vi "Run Post-Compile Hook.vi"(7 "Datum":refnum<class "Datum.lvclass">, 8 "Error In":errorcluster, 10 "Hooks In":T1, 11 "Output In":string) -> (0 "Error Out":errorcluster, 2 "Hooks Out":T1, 3 "Output Out":string)   [LabVIEW 2018, in "Toolkit.lvlib"]
uses:
  Toolkit.lvlib
  Low-Level/Type Definitions/Hooks.ctl
  Hooks/Compile/Process/Process.lvclass
  Hooks/Render/Comment/Comment.lvclass
  Hooks/Render/Delimiter/Delimiter.lvclass
  Hooks/Render/Node/Node.lvclass
  Hooks/Render/Partial/Partial.lvclass
  Hooks/Render/Process/Process.lvclass
  Hooks/Render/Section/Section.lvclass
  Hooks/Render/Text/Text.lvclass
  Hooks/Render/Variable/Variable.lvclass
  Data/Datum/Datum.lvclass
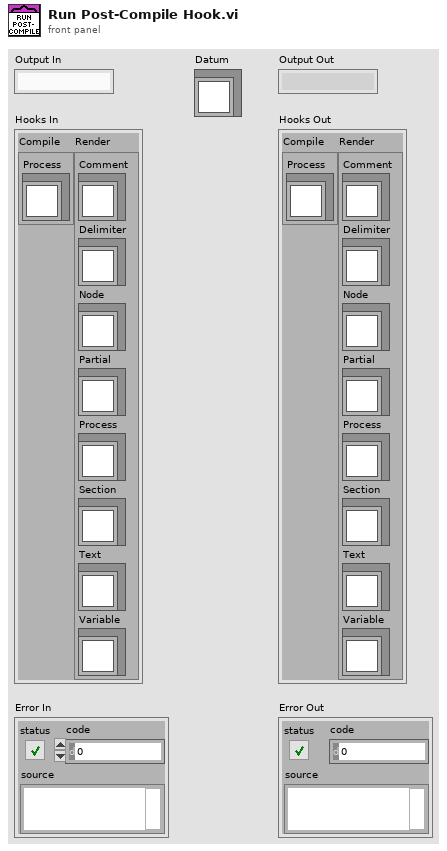
[diagram p1: front panel]
types:
  T1 = typedef "Toolkit.lvlib/Hooks.ctl" = cluster{"Compile":cluster{"Process":refnum<class "Process.lvclass">}, "Render":cluster{"Comment":refnum<class "Comment.lvclass">, "Delimiter":refnum<class "Delimiter.lvclass">, "Node":refnum<class "Node.lvclass">, "Partial":refnum<class "Partial.lvclass">, "Process":refnum<class "Process.lvclass">, "Section":refnum<class "Section.lvclass">, "Text":refnum<class "Text.lvclass">, "Variable":refnum<class "Variable.lvclass">}}
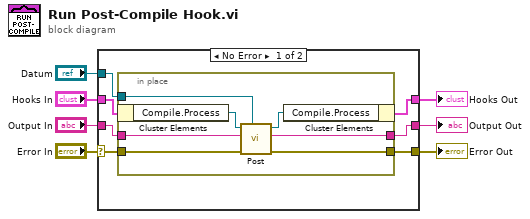
[diagram p0: block diagram]
diagram:
  n1 = case shown="No Error" "Error In" {
    selector: "Error In" -> [w13 w24]
    tunnel: [w12 w24] -> w7
    tunnel: "Hooks In" -> [w9 w22]
    tunnel: "Datum" -> [w14 _]
    tunnel: "Output In" -> [w11 w23]
    tunnel: [w10 w23] -> w2
    tunnel: [w8 w22] -> w1
    frame No Error {
      n2 = in-place {
        in-place-border: w14 -> [w21]
        in-place-border: w13 -> [w20]
        in-place-border: [w19] -> w12
        in-place-border: w11 -> [w18]
        in-place-border: [w17] -> w10
        n3 = in-place-cluster #1(w9) -> ("Compile.Process"=w16:refnum<class "Process.lvclass">)
        n4 = call-dynamic "Post.vi"("Datum"=w21, "Error In"=w20, "Output In"=w18, "Render In"=w16) -> ("Error Out"=w19:errorcluster, "Output Out"=w17:string, "Render Out"=w15:refnum<class "Process.lvclass">)  [unwired: 5 in]
        n5 = in-place-cluster #1("Compile.Process"=w15) -> (w8:T1)
      }
    }
    frame Error {
    }
  }
  "Error Out" <- w7
  "Output Out" <- w2
  "Hooks Out" <- w1
